vi "Write TemplatesFolder Key.vi"(8 "Error In":errorcluster, 11 "Templates Folder Path":string) -> (0 "Error Out":errorcluster)   [LabVIEW 2021]
doc: "<add documentation here>"
uses:
  <vilib>/registry/registry.llb/Write Registry Value Simple STR.vi
panel:
  # "Development\nControls or indicators that are useful for development or testing, but which are not outputs of the VI."
  # "Input\nInputs to the VI"
  # "Output\nOutputs of the VI"
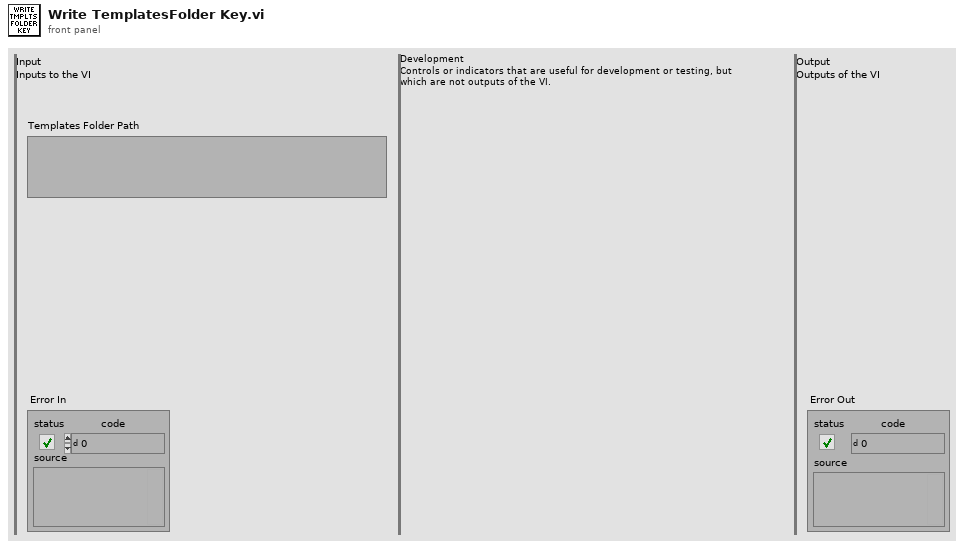
[diagram p1: front panel]
types:
  T1 = typedef "Registry RtKey.ctl" = enum32{"HKEY_CLASSES_ROOT", "HKEY_CURRENT_USER", "HKEY_LOCAL_MACHINE", "HKEY_USERS", "HKEY_PERFORMANCE_DATA", "HKEY_CURRENT_CONFIG", "HKEY_DYN_DATA"}
  T2 = typedef "Registry refnum.ctl" = refnum<k1>
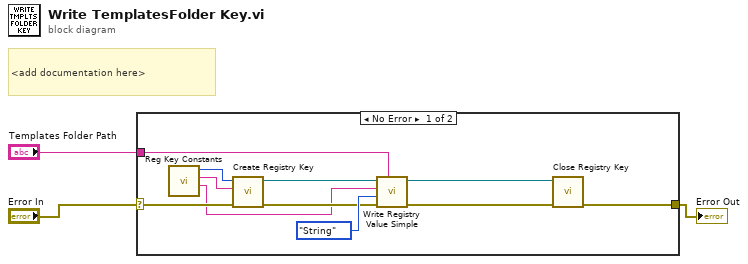
[diagram p0: block diagram]
diagram:
  # "<add documentation here>"
  n1 = case shown="No Error" "Error In" {
    selector: "Error In" -> [w9 w15]
    tunnel: [w6 w15] -> w2
    tunnel: "Templates Folder Path" -> [w5 _]
    frame No Error {
      n2 = call "Reg Key Constants.vi"() -> ("String Value Name"=w4:string, "Subkey Path"=w14:string, "Root Key"=w13:T1)  [unwired: 4 in, 1 out]
      n3 = call <vilib>:"Create Registry Key.vi"("error in (no error)"=w9, "subkey"=w14, "root key (HKEY_LOCAL_MACHINE)"=w13) -> ("error out"=w8:errorcluster, "refnum out"=w12:T2)  [unwired: 6 in, 1 out]
      n4 = call-poly <vilib>:"Write Registry Value Simple.vi"("String/Binary data"=w5, "error in (no error)"=w8, "simple data type"=enum16{"String", "Binary", "DWORD"}."String", "value"=w4, "refnum"=w12) -> ("error out"=w7:errorcluster, "refnum out"=w11:T2)  [unwired: 3 in]
      n5 = call <vilib>:"Close Registry Key.vi"("error in (no error)"=w7, "refnum"=w11) -> ("error out"=w6:errorcluster)  [unwired: 5 in]
    }
    frame Error {
    }
  }
  "Error Out" <- w2
